vi "new results.vi"(8 "error in (no error)":errorcluster, 9 "Results In":refnum<class "Analyze Results Base.lvclass">[](array[class]), 10 "Parameters":refnum<class "Analyze Parameter Base.lvclass">[](array[class]), 11 "Camera Display in":refnum<class "Camera Display.lvclass">) -> (0 "error out":errorcluster, 3 "Camera Display out":refnum<class "Camera Display.lvclass">)   [LabVIEW 2014, in "Camera Display.lvlib" / "Camera Display.lvclass"]
uses:
  Camera Display.lvclass
  Results and Overlays/Results Base/Analyze Results Base.lvclass
  Analyze Parameter/Analyze Parameter Base/Analyze Parameter Base.lvclass
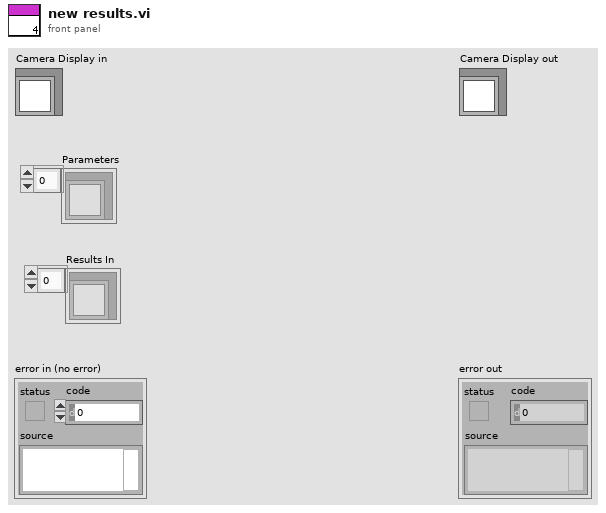
[diagram p1: front panel]
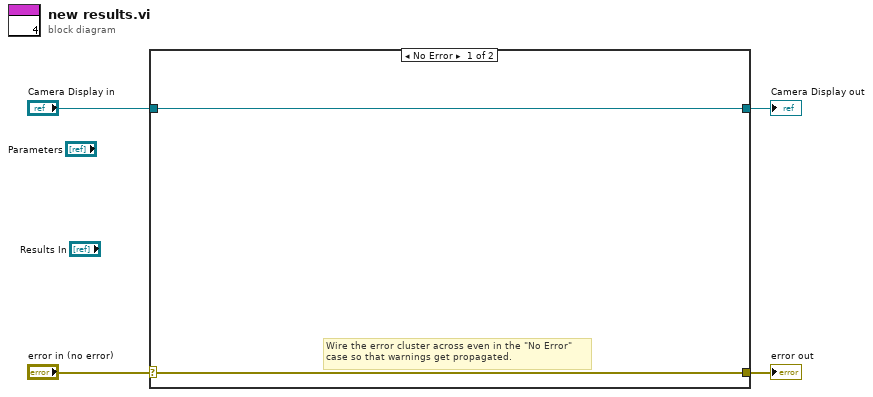
[diagram p0: block diagram]
diagram:
  n1 = case shown="No Error" "error in (no error)" {
    selector: "error in (no error)" -> [w5 w8]
    tunnel: [w5 w8] -> w3
    tunnel: [w6 w7] -> w1
    tunnel: "Camera Display in" -> [w6 w7]
    frame No Error {
      # "Wire the error cluster across even in the \"No Error\"\ncase so that warnings get propagated."
    }
    frame Error {
    }
  }
  "error out" <- w3
  "Camera Display out" <- w1
